vi "Handle Last Ack Core.vi"(4 "error in (no error)":errorcluster, 6 "Last Ack":refnum<class "Last Ack.lvclass">, 7 "Mediator in":refnum<class "Mediator.lvclass">) -> (0 "error out":errorcluster, 3 "Mediator out":refnum<class "Mediator.lvclass">)   [LabVIEW 2015, in "Mediator.lvlib" / "Mediator.lvclass"]
doc: "(<B>Filename</B>: Actor Framework.lvlib:Actor.lvclass:Handle Last Ack Core.vi)\n\nDefines how the caller actor responds to the Last Ack message from a nested actor. The Last Ack message is the final message a nested actor sends to its caller before it shuts down. The message contains information about the final state of the nested actor.\n\nBy default, this method does nothing except return any error the nested actor sent. A descendant class may override this method to define behavior.\n\n<License>\nCopyright © 2017 Composed Systems, LLC | All rights reserved\nwww.composed.io\n\nAuthor: Ethan Stern <ethan.stern@composed.io>\n\nThis software is provided \"AS IS\" WITHOUT WARRANTIES, either express or implied, AND IS FOR EDUCATIONAL PURPOSES ONLY.\n</License>"
uses:
  Mediator.lvclass
  <vilib>/ActorFramework/LastAck/Last Ack.lvclass
  Topic/Topic.lvclass
  <vilib>/ActorFramework/LastAck/Last Ack.lvclass/Last Ack.ctl
  Mediator.lvclass/Mediator.ctl
  TopicLookupTable/TopicLookupTable.lvclass
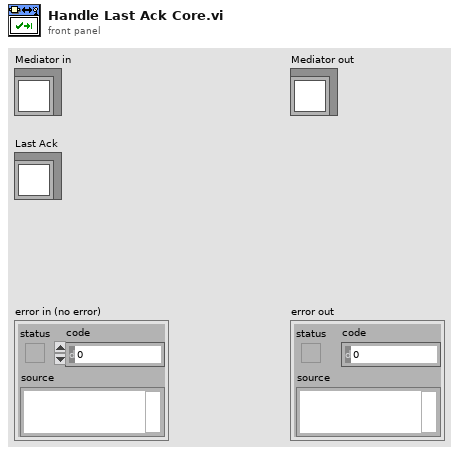
[diagram p1: front panel]
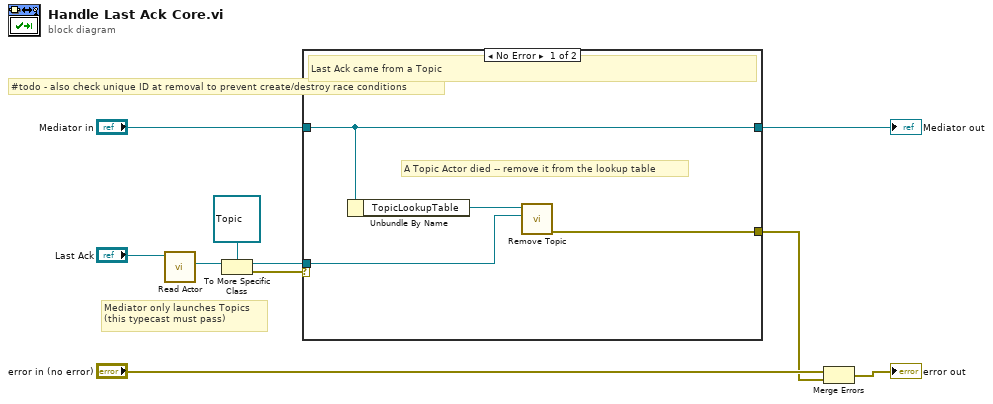
[diagram p0: block diagram]
diagram:
  # "#todo - also check unique ID at removal to prevent create/destroy race conditions"
  # "Mediator only launches Topics\n(this typecast must pass)"
  n1 = call <vilib>:"Read Actor.vi"("Last Ack"="Last Ack") -> ("Actor"=w8:refnum<class "Actor.lvclass">)  [unwired: 10 in]
  n2 = To More Specific Class(target class=refnum<class "Topic.lvclass"> refnum ("Mediator.lvlib:Topic.lvclass"), reference=w8) -> (specific class reference=w6:refnum<class "Topic.lvclass">, error out=w1:errorcluster)  [unwired: 1 in]
  n3 = case shown="No Error" w1 {
    selector: w1 -> [_ w15]
    tunnel: w6 -> [w14 _]
    tunnel: "Mediator in" -> [w13 w16]
    tunnel: [w13 w16] -> w4
    tunnel: [w12 w15] -> w2
    frame No Error {
      # "A Topic Actor died -- remove it from the lookup table"
      # "Last Ack came from a Topic"
      n4 = Unbundle By Name(w13) -> ("TopicLookupTable"=w11:refnum<data-value>)
      n5 = call "Remove Topic.vi"("Topic"=w14, "TopicLookupTable"=w11) -> ("error out"=w12:errorcluster)  [unwired: 8 in, 1 out]
    }
    frame Error {
      # "The typecast failed -- the sky is definitely falling"
    }
  }
  "Mediator out" <- w4
  n6 = Merge Errors("error in (no error)", w2) -> (→"error out":errorcluster)
